vi "Arrange Terminal Lookup.vi"(10 "Arrange":T1, 11 "Terminals":refnum<vi>[](array[refnum])) -> (3 "Terminal Index":i32)   [LabVIEW 2019, in "Builtins.lvlib"]
doc: "Returns the input or output terminal index using the terminal postion and Left-to-Right (L2R) or Right-to-Left (R2L) conditions:\n\nIF input count <= 0:\n L2R = bottom-right output term idx\n R2L = top-right output term idx\nELIF input count == 1:\n L2R =bottom-left input term idx\n R2L = bottom-right output term idx\nELIF input count >= 2 && output count <= 0:\n L2R = bottom-left input term idx\n R2L = top-left input term idx\nELIF input count >= 2 && output count >= 1:\n L2R = bottom-left input term idx\n R2L = bottom-right output term idx\n\nCreated by: Ryan Pacini"
uses:
  Builtins.lvlib
  Arrange.ctl
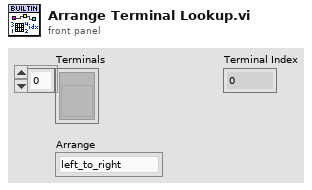
[diagram p1: front panel]
types:
  T1 = typedef "Builtins.lvlib/Arrange.ctl" = enum8{"left_to_right", "right_to_left"}
  T2 = typedef "LVRectTypeDef.ctl" = cluster{"Left":i16, "Top":i16, "Right":i16, "Bottom":i16}
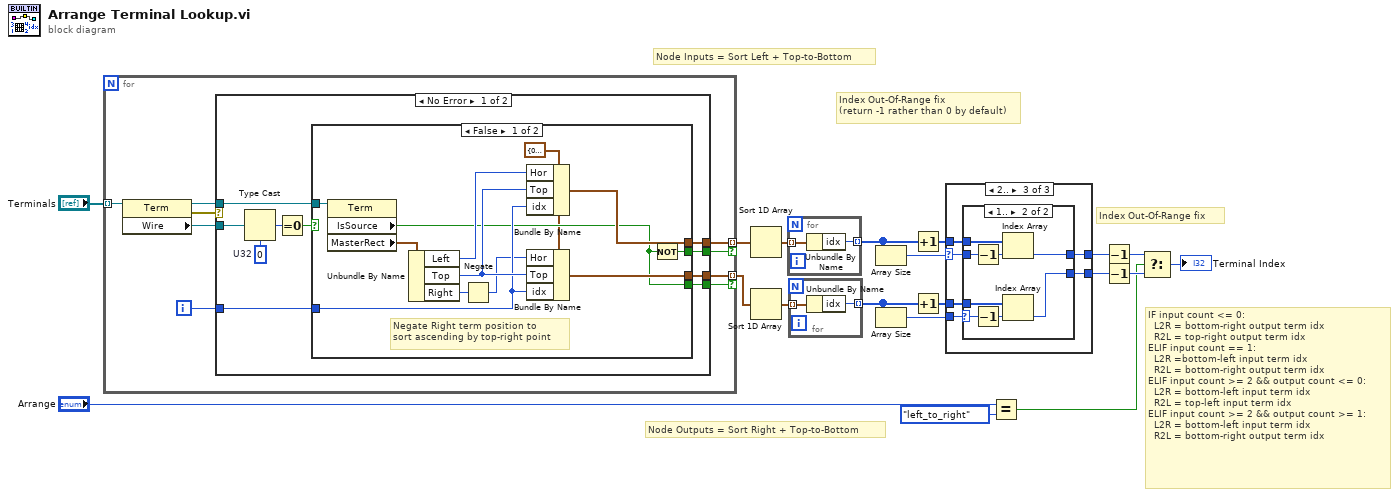
[diagram p0: block diagram]
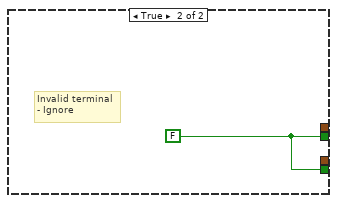
[diagram p2: hidden frame]
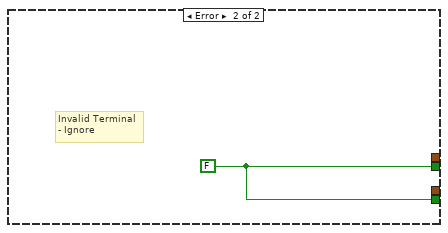
[diagram p3: hidden frame]
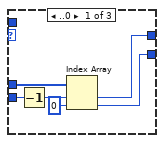
[diagram p4: hidden frame]
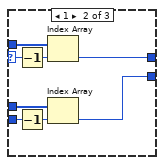
[diagram p5: hidden frame]
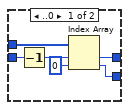
[diagram p6: hidden frame]
diagram:
  # "IF input count <= 0:\n  L2R = bottom-right output term idx\n  R2L = top-right output term idx\nELIF input count == 1:\n  L2R =bottom-left input term idx\n  R2L = bottom-right output term idx\nELIF input count >= 2 && output count <= 0:\n  L2R = bottom-left input term idx\n  R2L = top-left input term idx\nELIF input count >= 2 && output count >= 1:\n  L2R = bottom-left input term idx\n  R2L = bottom-right output term idx"
  # "Index Out-Of-Range fix"
  # "Index Out-Of-Range fix\n(return -1 rather than 0 by default)"
  # "Node Outputs = Sort Right + Top-to-Bottom"
  # "Node Inputs = Sort Left + Top-to-Bottom"
  n1 = for {
    tunnel: [w28] -> w19 mode=indexing if=w25
    tunnel: [w27] -> w18 mode=indexing if=w24
    tunnel: "Terminals" -> [w22] mode=indexing
    i -> [w26]
    n2 = property class="Term"(reference=w22) -> (reference out=w21:refnum<vi>, error out=w20:errorcluster, "Wire"=w23:refnum<vi>)  [unwired: 1 in]
    n3 = case shown="No Error" w20 {
      tunnel: [w38 _] -> w28
      tunnel: [w37 _] -> w27
      tunnel: w26 -> [w36 _]
      tunnel: [w35 w52] -> w25
      tunnel: [w34 w52] -> w24
      tunnel: w23 -> [w31 _]
      tunnel: w21 -> [w29 _]
      frame No Error {
        w33 = u32 0  # U32
        n4 = Type Cast(type=w33, x=w31) -> (*(type *) &x=w32:u32)
        n5 = Equal To 0?(x=w32) -> (x = 0?=w30:bool)
        n6 = case shown="False" w30 {
          tunnel: w29 -> [w50 _]
          tunnel: [w47 _] -> w38
          tunnel: [w46 _] -> w37
          tunnel: w36 -> [w44 _]
          tunnel: [w43 w51] -> w35
          tunnel: [w42 w51] -> w34
          frame False {
            w39 = cluster{"Top":i16, "Hor":i16, "idx":i32} {"Top"=0, "Hor"=0, "idx"=0} ("cluster")
            # "Negate Right term position to\nsort ascending by top-right point"
            n7 = property class="Term"(reference=w50) -> ("IsSource"=w42:bool, "MasterRect"=w49:T2)  [unwired: 1 in, 2 out]
            n8 = Unbundle By Name(w49) -> ("Left"=w48:i16, "Top"=w45:i16, "Right"=w41:i16)
            n9 = Negate(x=w41) -> (-x=w40:i16)
            n10 = Bundle By Name(cluster=w39, "Hor"=w48, "Top"=w45, "idx"=w44) -> (w47:cluster{"Top":i16, "Hor":i16, "idx":i32})
            n11 = Bundle By Name(cluster=w39, "Hor"=w40, "Top"=w45, "idx"=w44) -> (w46:cluster{"Top":i16, "Hor":i16, "idx":i32})
            n12 = Not(x=w42) -> (.not. x?=w43:bool)
          }
          frame True {
            w51 = FALSE
            # "Invalid terminal\n- Ignore"
          }
        }
      }
      frame Error {
        w52 = FALSE
        # "Invalid Terminal\n- Ignore"
      }
    }
  }
  n13 = Sort 1D Array(array=w19) -> (sorted array=w17:cluster{"Top":i16, "Hor":i16, "idx":i32}[])
  n14 = Sort 1D Array(array=w18) -> (sorted array=w16:cluster{"Top":i16, "Hor":i16, "idx":i32}[])
  n15 = for {
    tunnel: w17 -> [w54] mode=indexing
    tunnel: [w53] -> w14 mode=indexing
    n16 = Unbundle By Name(w54) -> ("idx"=w53:i32)
  }
  n17 = for {
    tunnel: w16 -> [w56] mode=indexing
    tunnel: [w55] -> w13 mode=indexing
    n18 = Unbundle By Name(w56) -> ("idx"=w55:i32)
  }
  n19 = Array Size(array=w14) -> (size(s)=w15:i32)
  n20 = Array Size(array=w13) -> (size(s)=w12:i32)
  n21 = Increment(x=w14) -> (x+1=w7:i32[])
  n22 = Increment(x=w13) -> (x+1=w8:i32[])
  n23 = case shown="2.." w15 {
    selector: w15 -> [_ w69 w74]
    tunnel: w7 -> [_ w70 w75]
    tunnel: w8 -> [w62 w65 w71]
    tunnel: w12 -> [w61 w64 w76]
    tunnel: [w58 w67 w73] -> w11
    tunnel: [w57 w63 w72] -> w10
    frame ..0 {
      n24 = Decrement(x=w61) -> (x-1=w60:i32)
      n25 = Index Array(array=w62, index #1=w60, index #2=0 ("index")) -> (element #1=w58:i32, element #2=w57:i32)
    }
    frame 1 {
      n26 = Decrement(x=w69) -> (x-1=w68:i32)
      n27 = Decrement(x=w64) -> (x-1=w66:i32)
      n28 = Index Array(array=w70, index=w68) -> (element=w67:i32)
      n29 = Index Array(array=w65, index=w66) -> (element=w63:i32)
    }
    frame 2.. {
      n30 = case shown="1.." w76 {
        selector: w76 -> [_ w84]
        tunnel: w75 -> [w82 w90]
        tunnel: w74 -> [w81 w89]
        tunnel: [w79 w87] -> w73
        tunnel: [w78 w83] -> w72
        tunnel: w71 -> [_ w85]
        frame ..0 {
          n31 = Decrement(x=w81) -> (x-1=w80:i32)
          n32 = Index Array(array=w82, index #1=w80, index #2=0 ("index")) -> (element #1=w79:i32, element #2=w78:i32)
        }
        frame 1.. {
          n33 = Decrement(x=w89) -> (x-1=w88:i32)
          n34 = Decrement(x=w84) -> (x-1=w86:i32)
          n35 = Index Array(array=w90, index=w88) -> (element=w87:i32)
          n36 = Index Array(array=w85, index=w86) -> (element=w83:i32)
        }
      }
    }
  }
  n37 = Equal?(x="Arrange", y=Arrange."left_to_right" ("Arrange")) -> (x = y?=w2:bool)
  n38 = Decrement(x=w11) -> (x-1=w6:i32)
  n39 = Decrement(x=w10) -> (x-1=w5:i32)
  n40 = Select(t=w6, s=w2, f=w5) -> (s? t:f=→"Terminal Index":i32)
